vi "Voltage and Current Ring Chooser.vi"(8 "error in (no error)":errorcluster, 11 "Yokogawa WT1600 in":refnum<class "Yokogawa WT1600.lvclass">) -> (0 "error out":errorcluster, 1 "Current Strings And Values []":T1, 2 "Voltage Strings And Values []":T1, 3 "Yokogawa WT1600 out":refnum<class "Yokogawa WT1600.lvclass">)   [LabVIEW 2013, in "Universal Power Meter.lvlib" / "Yokogawa WT1600.lvlib" / "Yokogawa WT1600.lvclass"]
uses:
  Yokogawa WT1600.lvclass
  <vilib>/Utility/miscctls.llb/LVStringsAndValuesArrayTypeDef_U16.ctl
panel:
  in  "A Range (9: 5A)":u16(ring)=9 items=["AUTO", "10 mA", "20 mA", "50 mA", "100 mA", "200 mA", "500 mA", "1 A", "2 A", "5 A", "10 A", "20 A", "50 A", "S-AUTO", "50 mV", "100 mV", "250 mV", "500 mV", "1 V", "2.5 V", "5 V", "10 V"]
  in  "V Range (12: 1000)":u16(ring)=12 items=["AUTO", "1.5", "3", "6", "10", "15", "30", "60", "100", "150", "300", "600", "1000"]
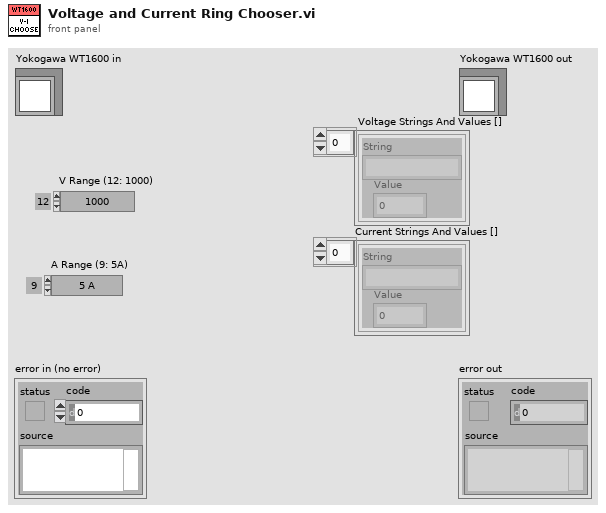
[diagram p1: front panel]
types:
  T1 = typedef "LVStringsAndValuesArrayTypeDef_U16.ctl" = cluster{"String":string, "Value":u16}[]
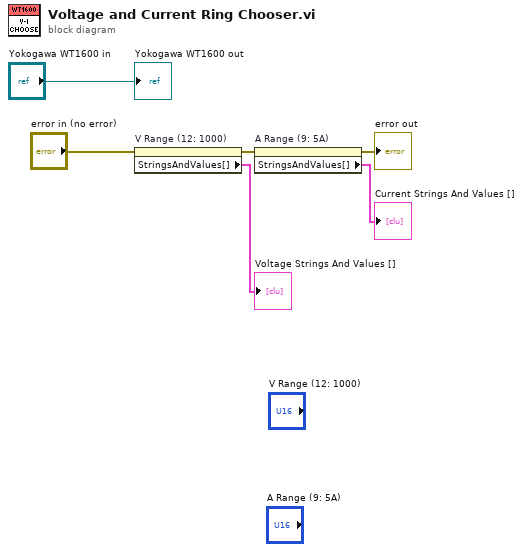
[diagram p0: block diagram]
diagram:
  n1 = property on="V Range (12: 1000)" class="Ring (strict)"(error in="error in (no error)") -> (error out=w5:errorcluster, "StringsAndValues[]"=→"Voltage Strings And Values []":T1)  [unwired: 1 in, 1 out]
  n2 = property on="A Range (9: 5A)" class="Ring (strict)"(error in=w5) -> (error out=→"error out":errorcluster, "StringsAndValues[]"=→"Current Strings And Values []":T1)  [unwired: 1 in, 1 out]
  "Yokogawa WT1600 out" <- "Yokogawa WT1600 in"
